vi "ScanDialog.vi"(8 "Error In":errorcluster, 9 "Channel Patterns":string[](array[string]), 10 "Slot Configuration":T1, 11 "Scan List In":string) -> (0 "Error Out":errorcluster, 2 "Cancelled?":bool, 3 "Scan List Out":string)   [LabVIEW 2012]
uses:
  SlotConfiguration.ctl
  BankConfiguration.ctl
  driver/Public/Controls/Slot.ctl
  libs/LV-Utilities/LV-Utilities.lvlib
  driver/Keithley-7001.lvlib
panel:
  in  "NEXT MEMORY LOCATION":bool
  in  "PREVIOUS MEMORY LOCATION":bool
  in  "Memory Location (1-100)":u8
  in  "ADD":bool
  out "Memory Channel Pattern":string
  out "Bank D Name":string
  out "Bank D Channel Names":string[](array[string])
  in  "Bank D Channel Enabled":bool[](array[boolean])
  out "Bank C Name":string
  out "Bank C Channel Names":string[](array[string])
  in  "Bank C Channel Enabled":bool[](array[boolean])
  out "Bank B Name":string
  out "Bank B Channel Names":string[](array[string])
  in  "Bank B Channel Enabled":bool[](array[boolean])=[FALSE, FALSE, FALSE, FALSE, FALSE, FALSE, FALSE, FALSE, FALSE, FALSE]
  out "Bank A Name":string
  out "Bank A Channel Names":string[](array[string])
  in  "Bank A Channel Enabled":bool[](array[boolean])=[FALSE, FALSE, FALSE, FALSE, FALSE, FALSE, FALSE, FALSE, FALSE, FALSE]
  in  "Scan List":string
  in  "RESET":bool
  in  "CANCEL":bool
  in  "DONE":bool
  # "MEMORY"
  # "Location"
  # "Channel Pattern"
  # "CHANNELS"
  # "Current Scan List"
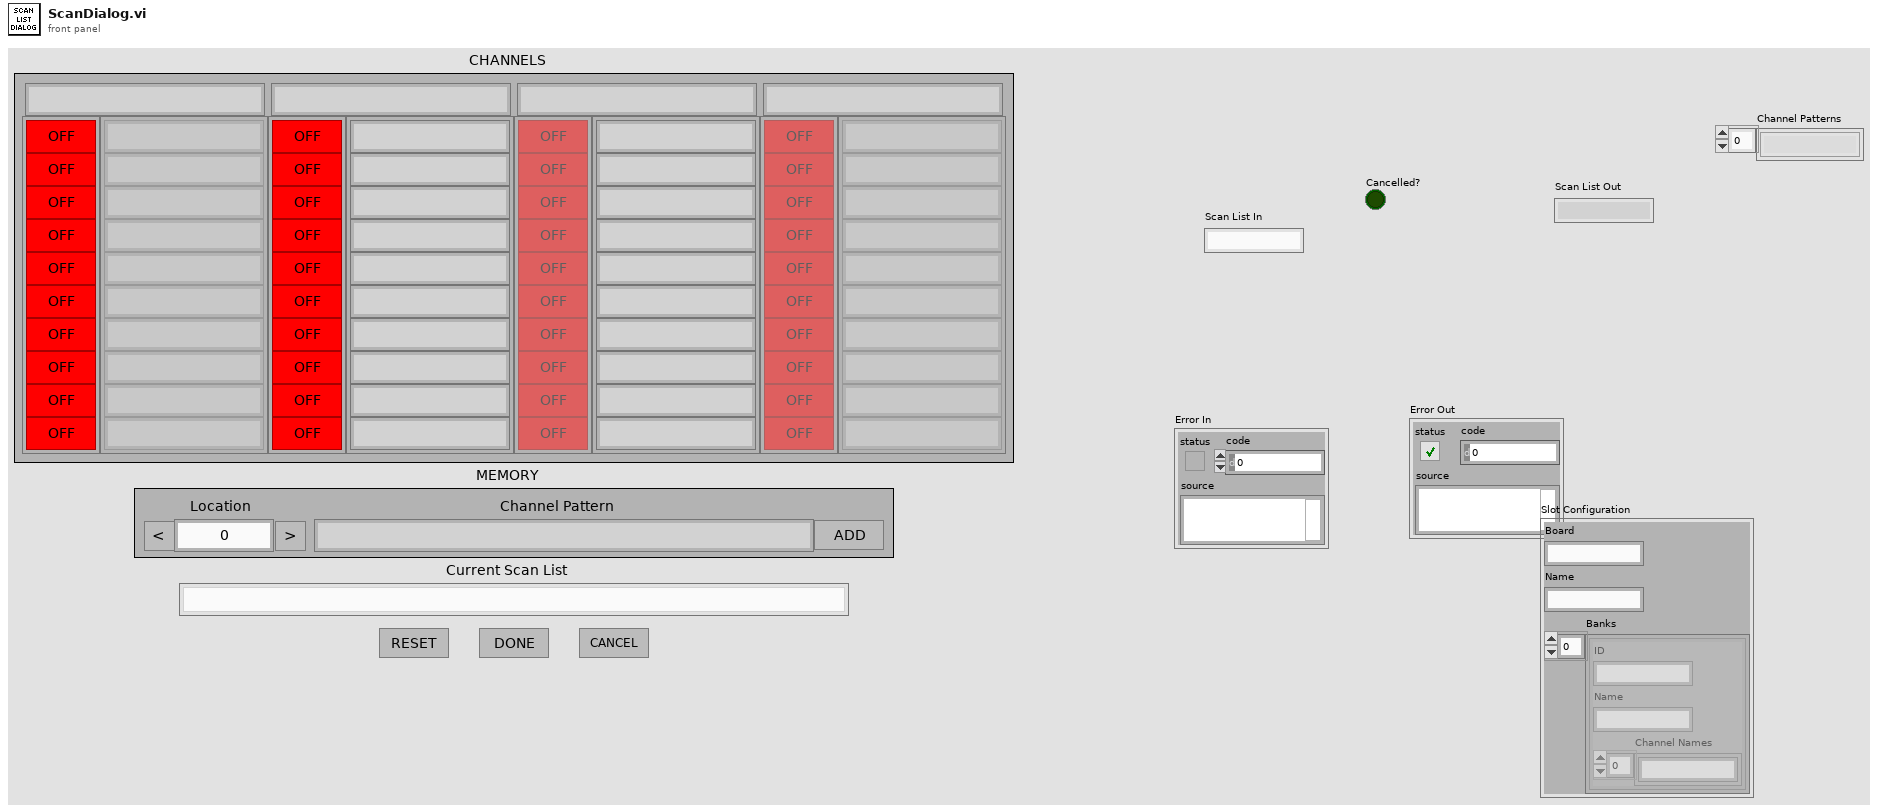
[diagram p1: front panel]
types:
  T1 = typedef "SlotConfiguration.ctl" = cluster{"Board":string, "Name":string, "Banks":T2[]}
  T2 = typedef "BankConfiguration.ctl" = cluster{"ID":string, "Name":string, "Channel Names":string[]}
  T3 = typedef "Keithley-7001.lvlib/Slot.ctl" = enum16{"Slot 1", "Slot 2"}
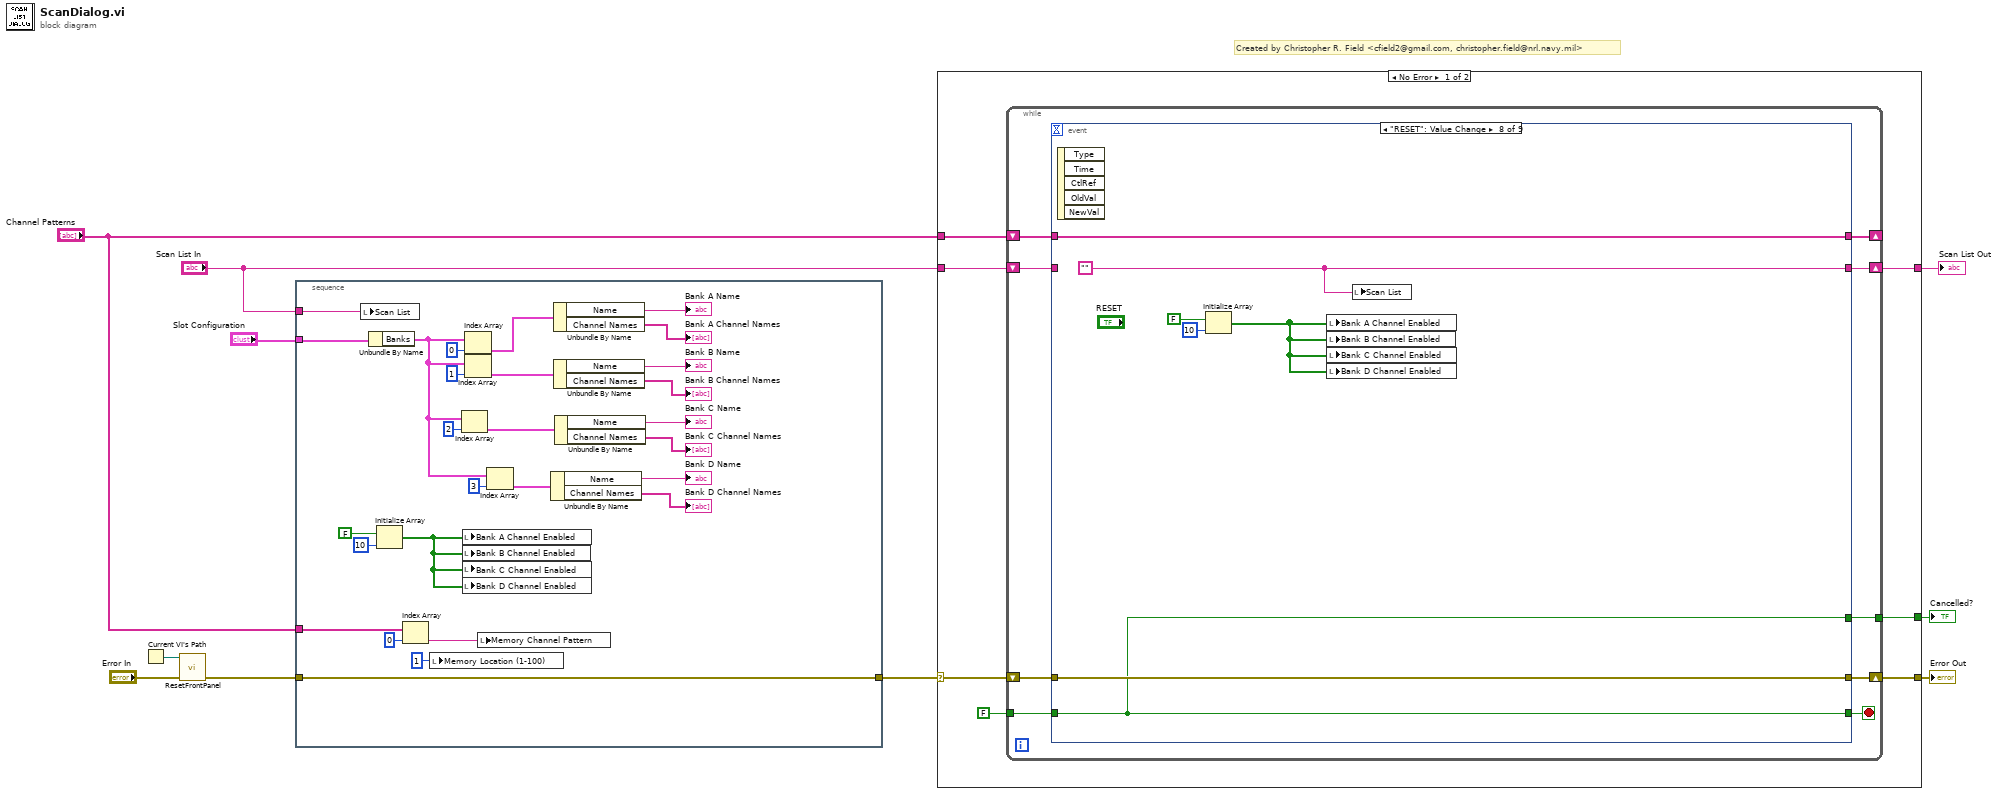
[diagram p0: block diagram]
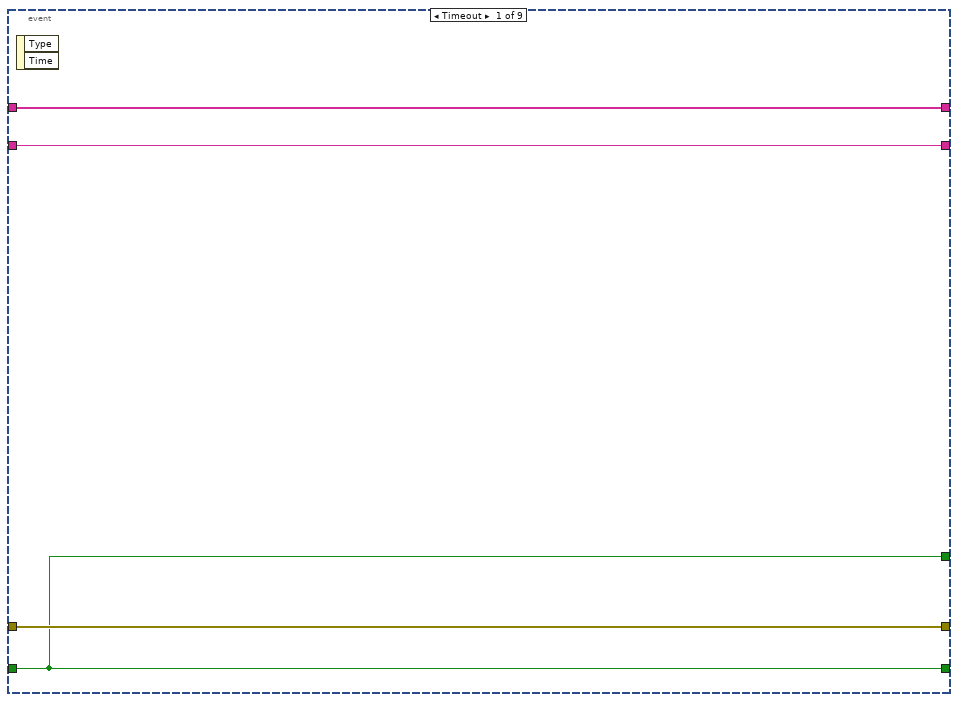
[diagram p2: hidden frame]
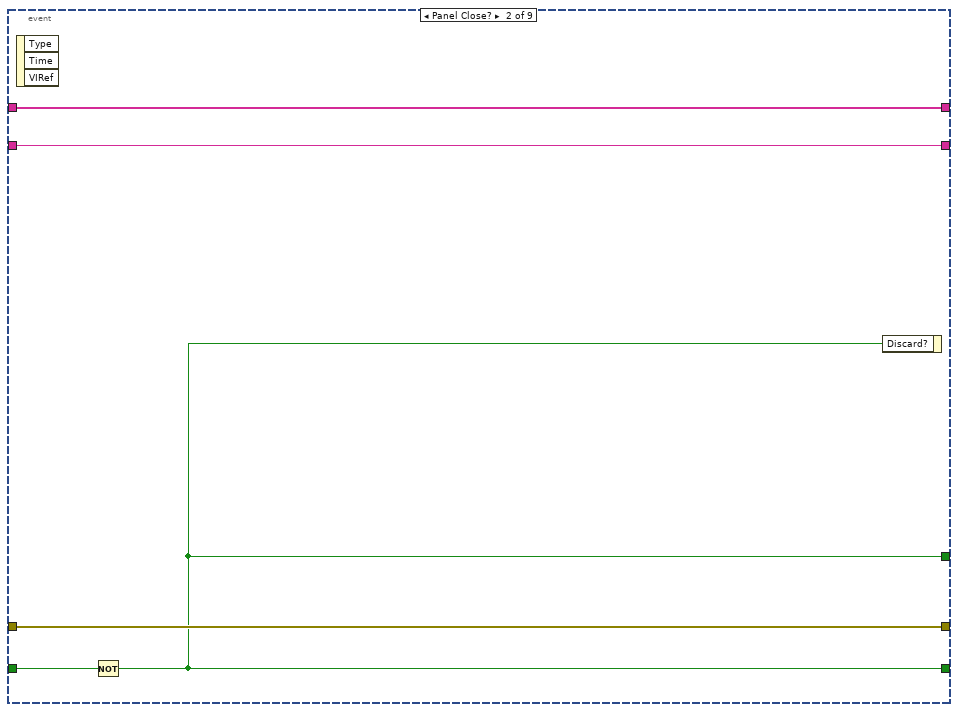
[diagram p3: hidden frame]
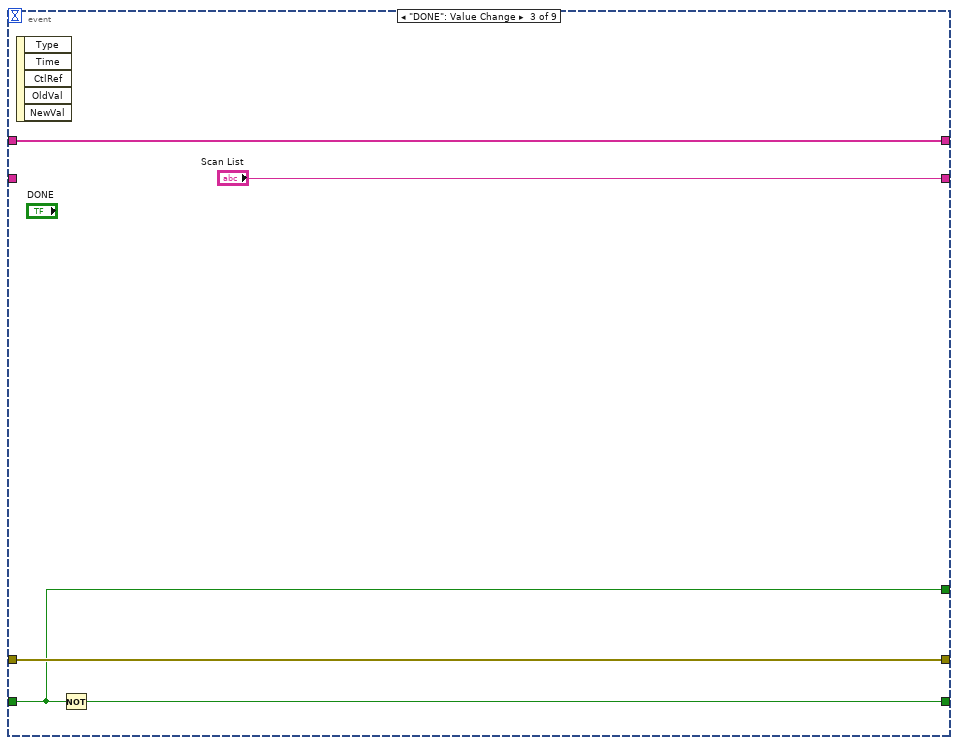
[diagram p4: hidden frame]
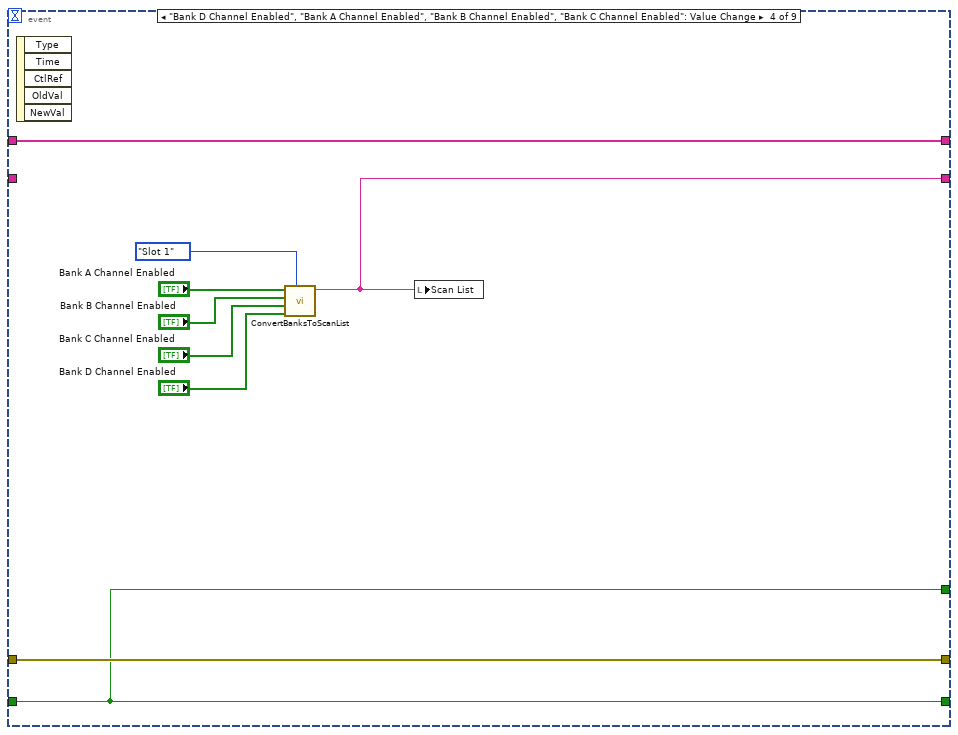
[diagram p5: hidden frame]
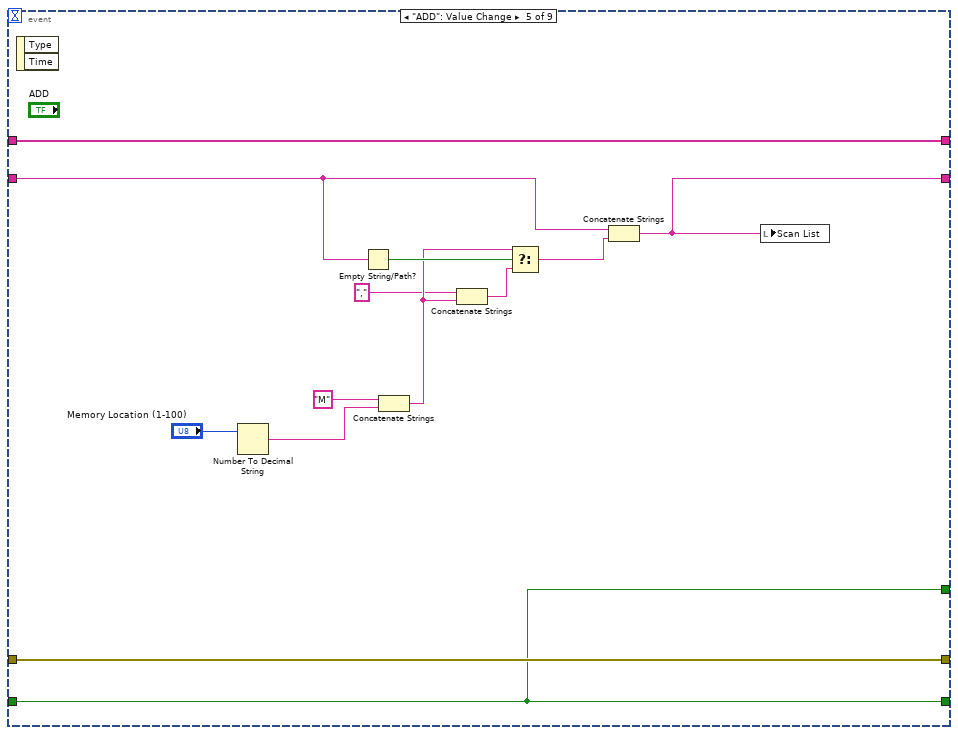
[diagram p6: hidden frame]
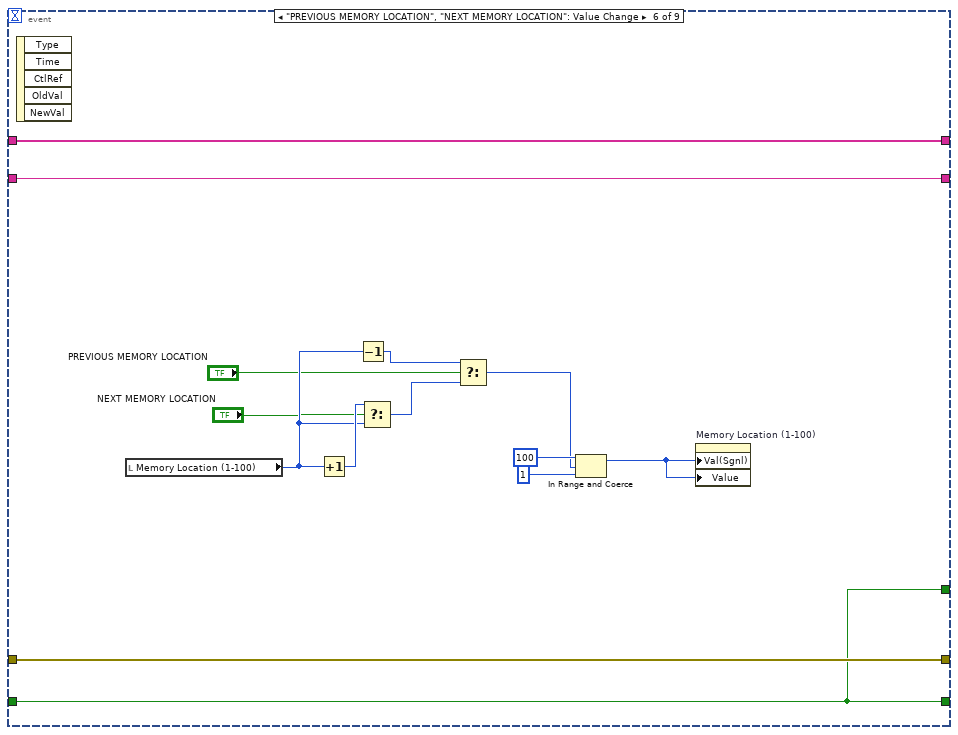
[diagram p7: hidden frame]
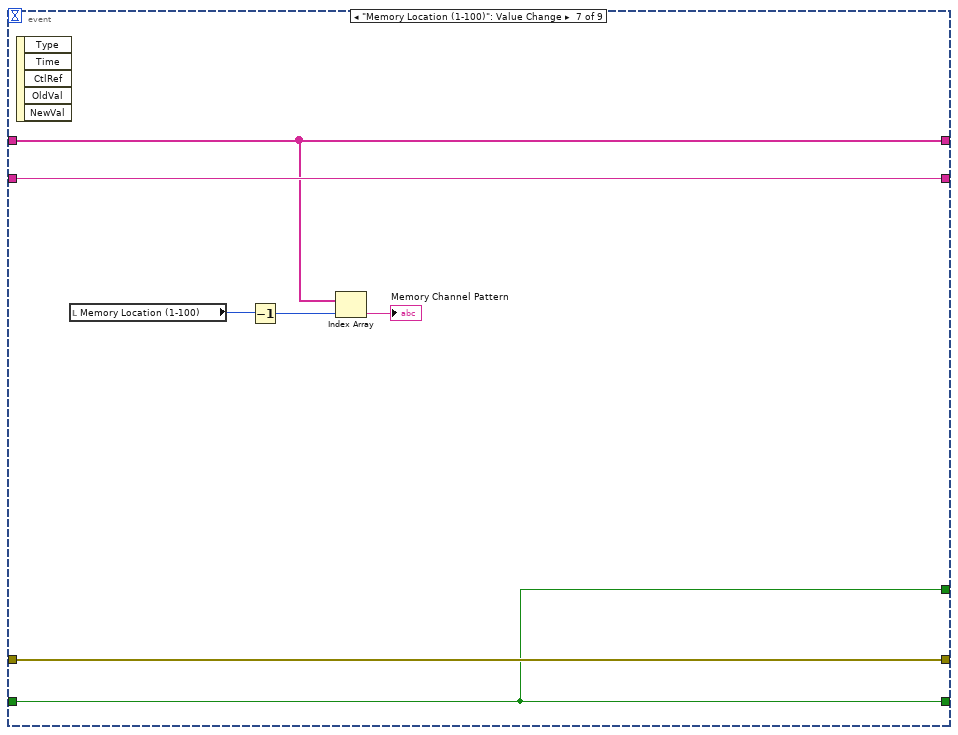
[diagram p8: hidden frame]
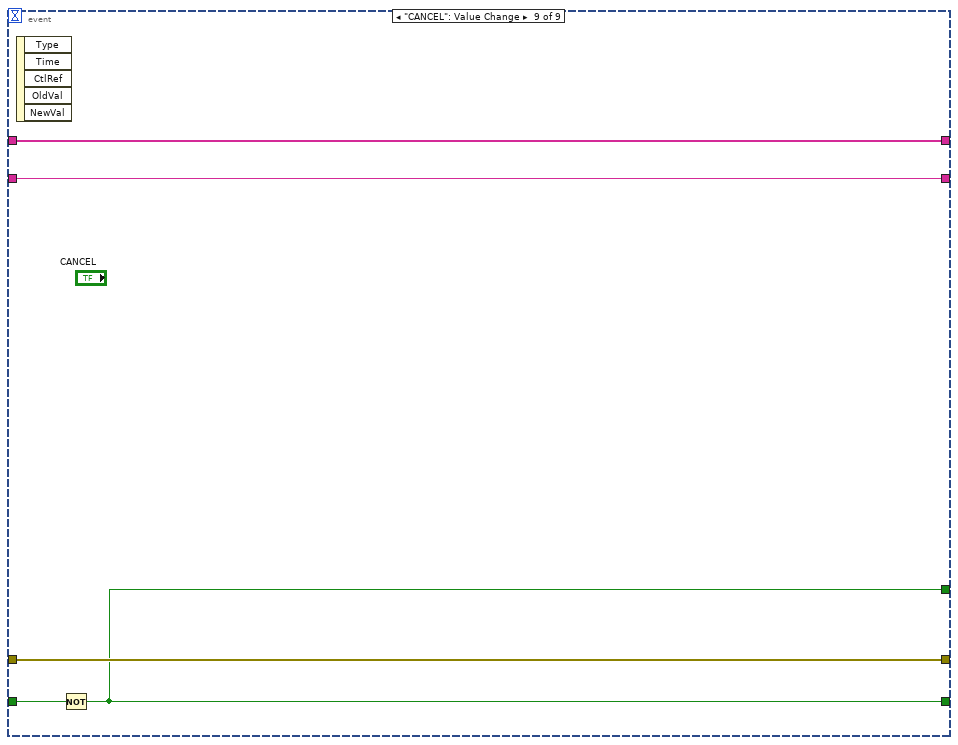
[diagram p9: hidden frame]
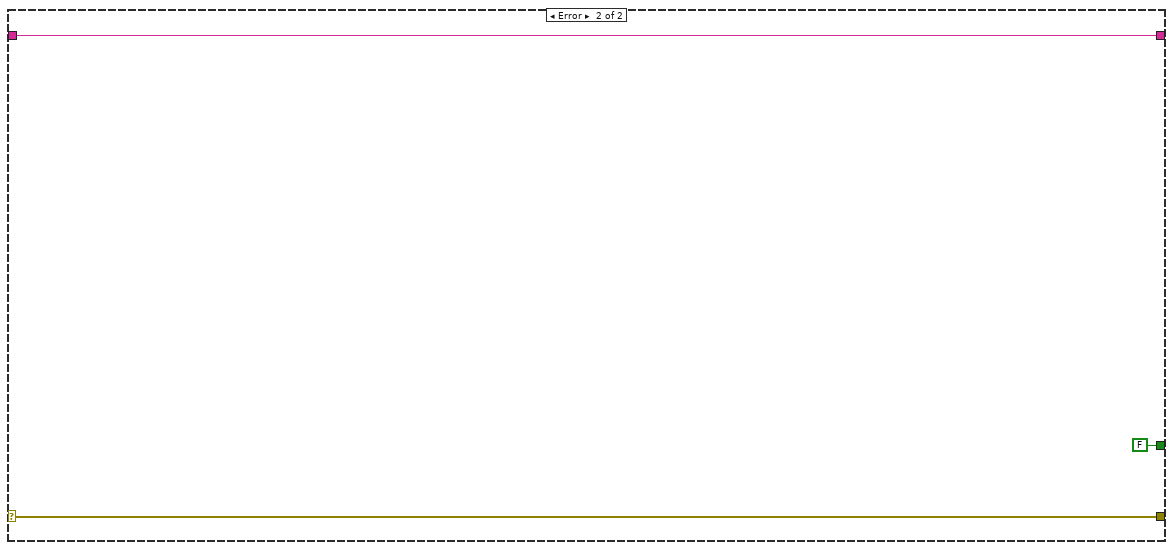
[diagram p10: hidden frame]
diagram:
  # "Created by Christopher R. Field <cfield2@gmail.com, christopher.field@nrl.navy.mil>"
  n1 = Current VI's Path() -> (path=w10:path)
  n2 = call "ResetFrontPanel.vi"("Error In"="Error In", "VI Path"=w10) -> ("Error Out"=w8:errorcluster)  [unwired: 9 in]
  n3 = stacked-sequence {
    tunnel: w8 -> [w37]
    tunnel: [w37] -> w7
    tunnel: "Scan List In" -> [w36]
    tunnel: "Slot Configuration" -> [w27]
    tunnel: "Channel Patterns" -> [w26]
    frame #0 {
      n4 = local write "Scan List"(w36) -> ()
      n5 = Unbundle By Name(w27) -> ("Banks"=w12:T2[])
      n6 = Initialize Array(FALSE, 10 ("dimension size")) -> (w20:bool[])
      n7 = Index Array(array=w26, index=0) -> (element=w24:string)
      n8 = local write "Memory Location (1-100)"(u8 1 ("Memory Location (1-100)")) -> ()
      n9 = Index Array(array=w12, index=2) -> (element=w13:T2)
      n10 = local write "Bank A Channel Enabled"(w20) -> ()
      n11 = local write "Bank B Channel Enabled"(w20) -> ()
      n12 = local write "Bank C Channel Enabled"(w20) -> ()
      n13 = local write "Bank D Channel Enabled"(w20) -> ()
      n14 = Index Array(array=w12, index=0) -> (element=w15:T2)
      n15 = Index Array(array=w12, index=1) -> (element=w14:T2)
      n16 = local write "Memory Channel Pattern"(w24) -> ()
      n17 = Index Array(array=w12, index=3) -> (element=w11:T2)
      n18 = Unbundle By Name(w11) -> ("Name"=→"Bank D Name":string, "Channel Names"=→"Bank D Channel Names":string[])
      n19 = Unbundle By Name(w15) -> ("Name"=→"Bank A Name":string, "Channel Names"=→"Bank A Channel Names":string[])
      n20 = Unbundle By Name(w14) -> ("Name"=→"Bank B Name":string, "Channel Names"=→"Bank B Channel Names":string[])
      n21 = Unbundle By Name(w13) -> ("Name"=→"Bank C Name":string, "Channel Names"=→"Bank C Channel Names":string[])
    }
  }
  n22 = case shown="No Error" w7 {
    selector: w7 -> [w44 w125]
    tunnel: [w42 w125] -> w6
    tunnel: [w41 FALSE] -> w5
    tunnel: "Scan List In" -> [w39 w123]
    tunnel: [w40 w123] -> w3
    tunnel: "Channel Patterns" -> [w38 _]
    frame No Error {
      n23 = while {
        tunnel: FALSE -> [w52]
        shift-right: [w50] -> w42
        shift-left: w44 -> [w53]
        tunnel: [w49] -> w41
        shift-right: [w48] -> w40
        shift-left: w39 -> [w47]
        shift-right: [w45] -> _
        shift-left: w38 -> [w46]
        stop <- w51 stop-if-true
        n24 = event shown="[7] \"RESET\": Value Change" {
          selector: _ -> [_ _ _ _ _ _ _ _ _]
          dyn-events: _ -> [_ _ _ _ _ _ _ _ _]
          timeout: _ -> [_ _ _ _ _ _ _ _ _]
          tunnel: w53 -> [w57 w62 w67 w76 w89 w95 w109 w117 w122]
          tunnel: w52 -> [w56 w61 w65 w75 w88 w94 w108 w116 w121]
          tunnel: [w56 w60 w66 w75 w88 w94 w108 w116 w120] -> w51
          tunnel: [w57 w62 w67 w76 w89 w95 w109 w117 w122] -> w50
          tunnel: [w56 w60 w65 w75 w88 w94 w108 w116 w120] -> w49
          tunnel: [w55 w59 "Scan List" w70 w77 w102 w110 w111 w119] -> w48
          tunnel: w47 -> [w55 w59 _ _ w79 w102 w110 _ w119]
          tunnel: w46 -> [w54 w58 w63 w68 w87 w103 w105 w115 w118]
          tunnel: [w54 w58 w63 w68 w87 w103 w105 w115 w118] -> w45
          event Timeout {
            n25 = event-data() -> ()  [unwired: 1 in, 2 out]
          }
          event Panel Close? {
            n26 = event-data() -> ()  [unwired: 1 in, 3 out]
            n27 = Not(x=w61) -> (.not. x?=w60:bool)
            n28 = event-data("Discard?"=w60) -> ()  [unwired: 1 in, 1 out]
          }
          event "DONE": Value Change {
            n29 = event-data() -> ()  [unwired: 1 in, 5 out]
            n30 = Not(x=w65) -> (.not. x?=w66:bool)
          }
          event "Bank D Channel Enabled", "Bank A Channel Enabled", "Bank B Channel Enabled", "Bank C Channel Enabled": Value Change {
            n31 = event-data() -> ()  [unwired: 1 in, 5 out]
            n32 = call "ConvertBanksToScanList.vi"("Slot"=Slot."Slot 1", "Bank D Channel Enabled"="Bank D Channel Enabled", "Bank C Channel Enabled"="Bank C Channel Enabled", "Bank B Channel Enabled"="Bank B Channel Enabled", "Bank A Channel Enabled"="Bank A Channel Enabled") -> ("Scan List"=w70:string)  [unwired: 6 in]
            n33 = local write "Scan List"(w70) -> ()
          }
          event "ADD": Value Change {
            n34 = event-data() -> ()  [unwired: 1 in, 2 out]
            n35 = Number To Decimal String(number="Memory Location (1-100)") -> (decimal integer string=w84:string)  [unwired: 1 in]
            n36 = Empty String/Path?(string/path=w79) -> (empty?=w83:bool)
            n37 = Concatenate Strings("M" ("string"), w84) -> (w82:string)
            n38 = Concatenate Strings("," ("string"), w82) -> (w80:string)
            n39 = Select(t=w82, s=w83, f=w80) -> (s? t:f=w78:string)
            n40 = Concatenate Strings(w79, w78) -> (w77:string)
            n41 = local write "Scan List"(w77) -> ()
          }
          event "PREVIOUS MEMORY LOCATION", "NEXT MEMORY LOCATION": Value Change {
            n42 = event-data() -> ()  [unwired: 1 in, 5 out]
            n43 = local read "Memory Location (1-100)"() -> (w93:u8)
            n44 = Increment(x=w93) -> (x+1=w99:u8)
            n45 = Decrement(x=w93) -> (x-1=w97:u8)
            n46 = Select(t=w99, s="NEXT MEMORY LOCATION", f=w93) -> (s? t:f=w98:u8)
            n47 = Select(t=w97, s="PREVIOUS MEMORY LOCATION", f=w98) -> (s? t:f=w96:u8)
            n48 = In Range and Coerce(upper limit=u8 100, x=w96, lower limit=u8 1) -> (coerced(x)=w90:u8)  [unwired: 1 out]
            n49 = property on="Memory Location (1-100)" class="DigNum (strict)"("Val(Sgnl)"=w90, "Value"=w90) -> ()  [unwired: 2 in, 2 out]
          }
          event "Memory Location (1-100)": Value Change {
            n50 = event-data() -> ()  [unwired: 1 in, 5 out]
            n51 = local read "Memory Location (1-100)"() -> (w107:u8)
            n52 = Decrement(x=w107) -> (x-1=w106:u8)
            n53 = Index Array(array=w105, index=w106) -> (element=→"Memory Channel Pattern":string)
          }
          event "RESET": Value Change {
            w111 = ""
            n54 = event-data() -> ()  [unwired: 1 in, 5 out]
            n55 = Initialize Array(FALSE, 10 ("dimension size")) -> (w112:bool[])
            n56 = local write "Bank A Channel Enabled"(w112) -> ()
            n57 = local write "Bank B Channel Enabled"(w112) -> ()
            n58 = local write "Bank C Channel Enabled"(w112) -> ()
            n59 = local write "Bank D Channel Enabled"(w112) -> ()
            n60 = local write "Scan List"(w111) -> ()
          }
          event "CANCEL": Value Change {
            n61 = event-data() -> ()  [unwired: 1 in, 5 out]
            n62 = Not(x=w121) -> (.not. x?=w120:bool)
          }
        }
      }
    }
    frame Error {
    }
  }
  "Error Out" <- w6
  "Cancelled?" <- w5
  "Scan List Out" <- w3
